vi "键盘.vi"(11 "原值":dbl) -> (3 "x+y":dbl format="%#_12g")   [LabVIEW 2013]
panel:
  in  "-":bool
  in  "清除":bool
  in  "退格":bool
  in  "取消按钮":bool
  in  ".":bool
  out "字符串":string
  in  "0":bool
  in  "停止":bool
  in  "9":bool
  in  "8":bool
  in  "7":bool
  in  "6":bool
  in  "5":bool
  in  "4":bool
  in  "3":bool
  in  "2":bool
  in  "1":bool
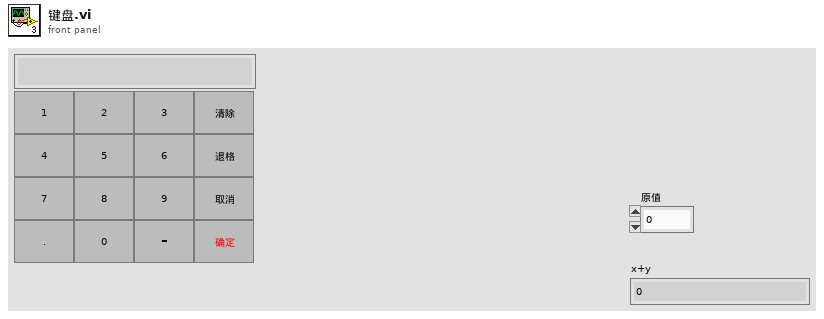
[diagram p1: front panel]
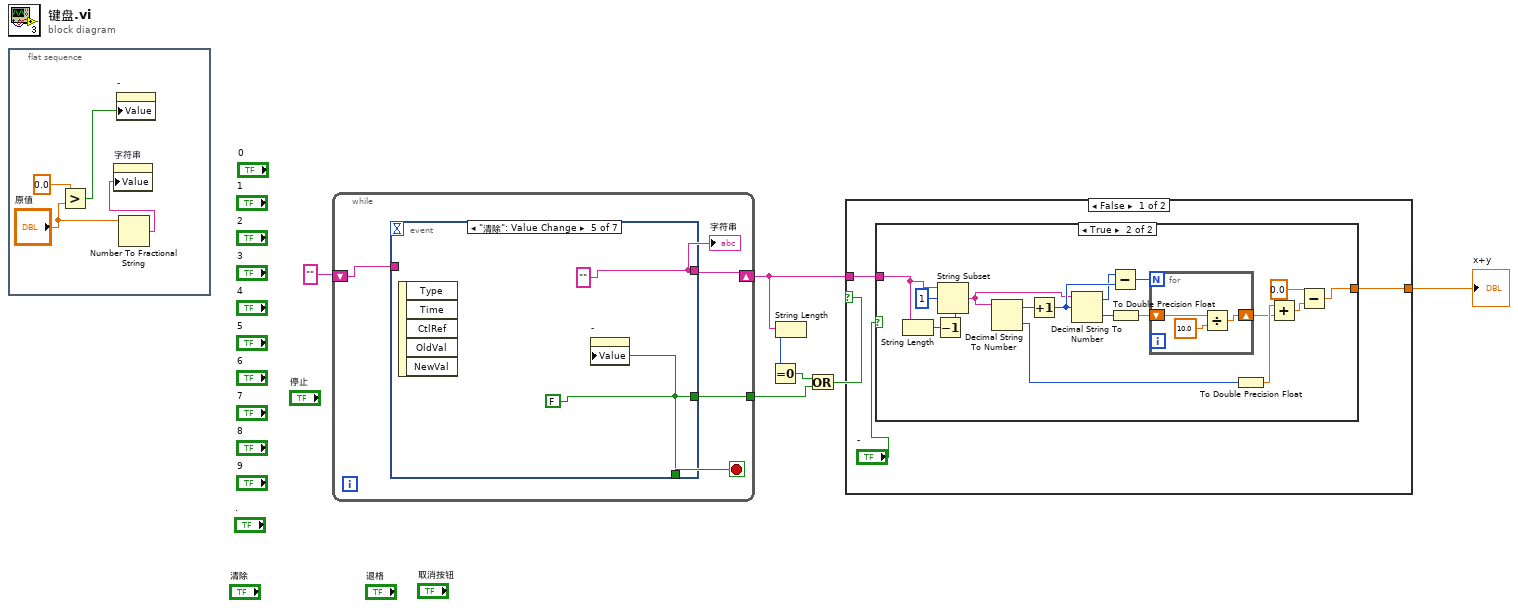
[diagram p0: block diagram]
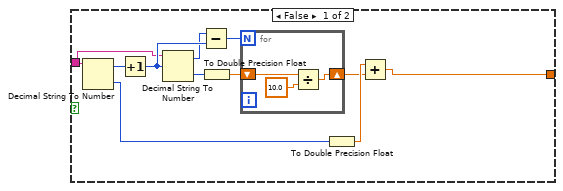
[diagram p2: hidden frame]
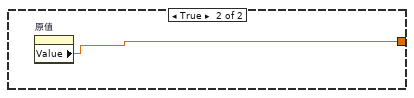
[diagram p3: hidden frame]
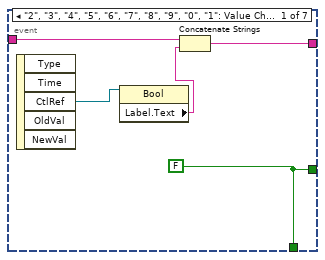
[diagram p4: hidden frame]
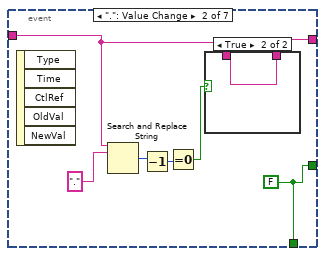
[diagram p5: hidden frame]
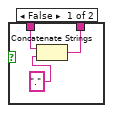
[diagram p6: hidden frame]
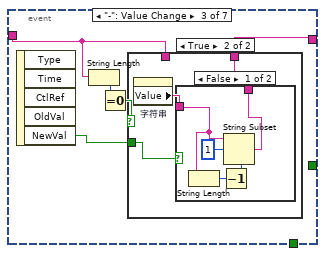
[diagram p7: hidden frame]
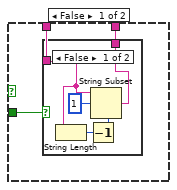
[diagram p8: hidden frame]
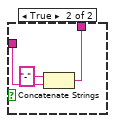
[diagram p9: hidden frame]
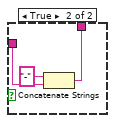
[diagram p10: hidden frame]
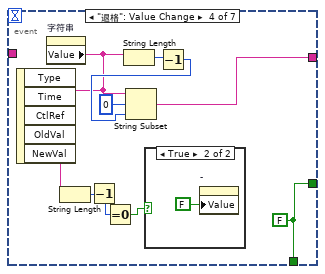
[diagram p11: hidden frame]
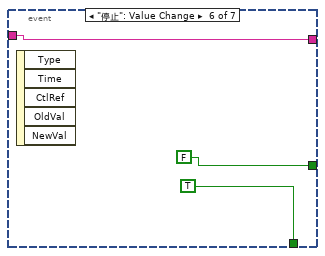
[diagram p13: hidden frame]
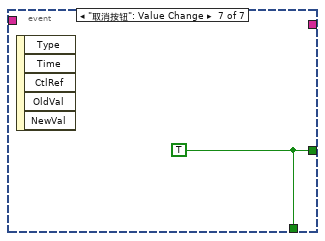
[diagram p14: hidden frame]
diagram:
  n1 = flat-sequence {
    frame #0 {
      n2 = Greater?(x=0.0, y="原值") -> (0:w8:bool)
      n3 = property on="-" class="Bool (strict)"("Value"=w8) -> ()  [unwired: 2 in, 2 out]
      n4 = Number To Fractional String(number="原值") -> (F-format string=w11:string)  [unwired: 3 in]
      n5 = property on="字符串" class="Str"("Value"=w11) -> ()  [unwired: 2 in, 2 out]
    }
  }
  n6 = while {
    shift-right: [w12] -> w6
    shift-left: "" ("Label.Text") -> [w14]
    tunnel: [w13] -> w1
    stop <- w15 stop-if-true
    n7 = event shown="[4] \"清除\": Value Change" {
      selector: _ -> [_ _ _ _ _ _ _]
      dyn-events: _ -> [_ _ _ _ _ _ _]
      timeout: _ -> [_ _ _ _ _ _ _]
      tunnel: [w16 w27 _ w63 w69 TRUE w74] -> w15
      tunnel: [w19 w22 w36 w64 "" ("Label.Text") w72 _] -> w12
      tunnel: w14 -> [w17 w21 w35 _ _ w72 _]
      tunnel: [w16 w27 _ w63 w69 FALSE w74] -> w13
      event "2", "3", "4", "5", "6", "7", "8", "9", "0", "1": Value Change {
        w16 = FALSE
        n8 = event-data() -> ("CtlRef"=w20:refnum<vi>)  [unwired: 1 in, 4 out]
        n9 = property class="Bool"(reference=w20) -> ("Label.Text"=w18:string)  [unwired: 1 in, 2 out]
        n10 = Concatenate Strings(w17, w18) -> (w19:string)
      }
      event ".": Value Change {
        w27 = FALSE
        n11 = event-data() -> ()  [unwired: 1 in, 5 out]
        n12 = Search and Replace String(input string=w21, search string="." ("搜索字符串")) -> (number of replacements=w26:i32)  [unwired: 6 in, 3 out]
        n13 = Decrement(x=w26) -> (x-1=w25:i32)
        n14 = Equal To 0?(x=w25) -> (x = 0?=w23:bool)
        n15 = case shown="True" w23 {
          tunnel: [w28 w31] -> w22
          tunnel: w21 -> [w29 w31]
          frame False {
            n16 = Concatenate Strings(w29, "." ("搜索字符串")) -> (w28:string)
          }
          frame True {
          }
        }
      }
      event "-": Value Change {
        n17 = event-data() -> ("NewVal"=w32:bool)  [unwired: 1 in, 4 out]
        n18 = String Length(string=w35) -> (length=w34:i32)
        n19 = Equal To 0?(x=w34) -> (x = 0?=w33:bool)
        n20 = case shown="True" w33 {
          tunnel: w35 -> [w39 _]
          tunnel: [w38 w48] -> w36
          tunnel: w32 -> [w37 w49]
          frame False {
            n21 = case shown="False" w37 {
              tunnel: w39 -> [w43 w47]
              tunnel: [w40 w46] -> w38
              frame False {
                n22 = String Length(string=w43) -> (length=w42:i32)
                n23 = Decrement(x=w42) -> (x-1=w41:i32)
                n24 = String Subset(string=w43, offset (0)=1 ("偏移量(0)"), length (rest)=w41) -> (substring=w40:string)
              }
              frame True {
                n25 = Concatenate Strings("-" ("字符串"), w47) -> (w46:string)
              }
            }
          }
          frame True {
            n26 = property on="字符串" class="Str"() -> ("Value"=w50:string)  [unwired: 2 in, 2 out]
            n27 = case shown="False" w49 {
              tunnel: w50 -> [w54 w58]
              tunnel: [w51 w57] -> w48
              frame False {
                n28 = String Length(string=w54) -> (length=w53:i32)
                n29 = Decrement(x=w53) -> (x-1=w52:i32)
                n30 = String Subset(string=w54, offset (0)=1 ("偏移量(0)"), length (rest)=w52) -> (substring=w51:string)
              }
              frame True {
                n31 = Concatenate Strings("-" ("字符串"), w58) -> (w57:string)
              }
            }
          }
        }
      }
      event "退格": Value Change {
        w63 = FALSE
        n32 = event-data() -> ()  [unwired: 1 in, 5 out]
        n33 = property on="字符串" class="Str"() -> ("Value"=w62:string)  [unwired: 2 in, 2 out]
        n34 = String Length(string=w62) -> (length=w61:i32)
        n35 = Decrement(x=w61) -> (x-1=w59:i32)
        n36 = Equal To 0?(x=w59) -> (x = 0?=w60:bool)
        n37 = String Length(string=w62) -> (length=w67:i32)
        n38 = case shown="True" w60 {
          frame False {
          }
          frame True {
            n39 = property on="-" class="Bool (strict)"("Value"=FALSE ("-")) -> ()  [unwired: 2 in, 2 out]
          }
        }
        n40 = Decrement(x=w67) -> (x-1=w65:i32)
        n41 = String Subset(string=w62, offset (0)=0 ("偏移量(0)"), length (rest)=w65) -> (substring=w64:string)
      }
      event "清除": Value Change {
        w69 = FALSE
        n42 = event-data() -> ()  [unwired: 1 in, 5 out]
        n43 = property on="-" class="Bool (strict)"("Value"=w69) -> ()  [unwired: 2 in, 2 out]
      }
      event "停止": Value Change {
        n44 = event-data() -> ()  [unwired: 1 in, 5 out]
      }
      event "取消按钮": Value Change {
        w74 = TRUE
        n45 = event-data() -> ()  [unwired: 1 in, 5 out]
      }
    }
    "字符串" <- w12
  }
  n46 = String Length(string=w6) -> (length=w5:i32)
  n47 = Equal To 0?(x=w5) -> (x = 0?=w4:bool)
  n48 = Or(x=w4, y=w1) -> (x .or. y?=w3:bool)
  n49 = case shown="False" w3 {
    tunnel: w6 -> [w77 _]
    tunnel: [w76 w112] -> w2
    frame False {
      n50 = case shown="True" "-" {
        tunnel: w77 -> [w79 w105]
        tunnel: [w78 w92] -> w76
        frame False {
          n51 = Decimal String To Number(string=w79) -> (offset past number=w88:i32, number=w87:i32)  [unwired: 2 in]
          n52 = Increment(x=w88) -> (x+1=w86:i32)
          n53 = Decimal String To Number(string=w79, offset=w86) -> (offset past number=w80:i32, number=w81:i32)  [unwired: 1 in]
          n54 = Subtract(x=w80, y=w86) -> (x-y=w85:i32)
          n55 = To Double Precision Float(number=w81) -> (double precision float=w84:dbl)
          n56 = for {
            N: w85 -> [_]
            shift-right: [w89] -> w82
            shift-left: w84 -> [w91]
            n57 = Divide(x=w91, y=sgl 10.0) -> (x/y=w89:dbl)
          }
          n58 = To Double Precision Float(number=w87) -> (double precision float=w83:dbl)
          n59 = Add(x=w83, y=w82) -> (x+y=w78:dbl)
        }
        frame True {
          n60 = String Length(string=w105) -> (length=w107:i32)
          n61 = Decrement(x=w107) -> (x-1=w106:i32)
          n62 = String Subset(string=w105, offset (0)=1 ("偏移量(0)"), length (rest)=w106) -> (substring=w95:string)
          n63 = Decimal String To Number(string=w95) -> (offset past number=w104:i32, number=w103:i32)  [unwired: 2 in]
          n64 = Increment(x=w104) -> (x+1=w102:i32)
          n65 = Decimal String To Number(string=w95, offset=w102) -> (offset past number=w96:i32, number=w97:i32)  [unwired: 1 in]
          n66 = Subtract(x=w96, y=w102) -> (x-y=w101:i32)
          n67 = To Double Precision Float(number=w97) -> (double precision float=w100:dbl)
          n68 = for {
            N: w101 -> [_]
            shift-right: [w109] -> w98
            shift-left: w100 -> [w111]
            n69 = Divide(x=w111, y=sgl 10.0) -> (x/y=w109:dbl)
          }
          n70 = To Double Precision Float(number=w103) -> (double precision float=w99:dbl)
          n71 = Add(x=w99, y=w98) -> (x+y=w94:dbl)
          n72 = Subtract(x=0.0, y=w94) -> (x-y=w92:dbl)
        }
      }
    }
    frame True {
      n73 = property on="原值" class="DigNum (strict)"() -> ("Value"=w112:dbl)  [unwired: 2 in, 2 out]
    }
  }
  "x+y" <- w2
